vi "Heading_Coor.vi"(10 "Azimuth Initial":dbl, 11 "heading (degrees)":dbl) -> (3 "Heading Coor":dbl)   [LabVIEW 2019]
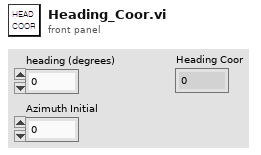
[diagram p1: front panel]
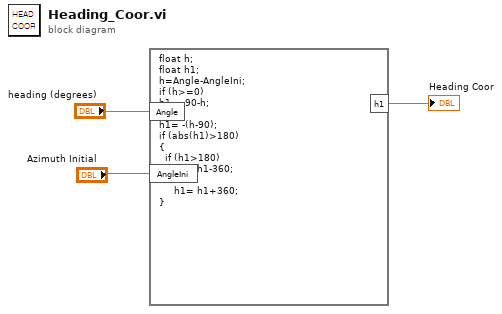
[diagram p0: block diagram]
diagram:
  n1 = formula code="float h;\nfloat h1;\nh=Angle-AngleIni;\nif (h>=0)\nh1 = 90-h;\nelse\nh1= -(h-90);\nif (abs(h1)>180)\n{\n  if (h1>180)\n     h1= h1-360;\n   else \n     h1= h1+360;\n}"("Angle"="heading (degrees)", "AngleIni"="Azimuth Initial") -> ("h1"=→"Heading Coor":dbl)
